vi "sv_Get Continuous Swept Sine Settings (1 Ch).vi"(8 "error in (no error)":errorcluster, 10 "chirp settings in":T1 {"frequency slope" format="%.2f"; "prefix len [samples]"."fractional" format="%.2p"; "initial states"."elapsed time [s]" format="%.2f"; "initial states"."phase [rad]" format="%.2f"; "initial states"."frequency [Hz]" format="%.2f"; "sampling info"."chirp duration [s]" format="%.2f"; "sampling info"."Fs" format="%.2p"; "frequency range"."stop (Hz)" format="%.2f"; "frequency range"."start (Hz)" format="%.2f"; "amplitude" format="%.2f"}, 11 "waveform":waveform(dbl)) -> (0 "error out":errorcluster, 2 "chirp settings out":T1 {"frequency slope" format="%.2f"; "prefix len [samples]"."fractional" format="%.2p"; "initial states"."elapsed time [s]" format="%.2f"; "initial states"."phase [rad]" format="%.2f"; "initial states"."frequency [Hz]" format="%.2f"; "sampling info"."chirp duration [s]" format="%.2f"; "sampling info"."Fs" format="%.2p"; "frequency range"."stop (Hz)" format="%.2f"; "frequency range"."start (Hz)" format="%.2f"; "amplitude" format="%.2f"}, 3 "same waveform":waveform(dbl))   [LabVIEW 2017]
uses:
  <vilib>/addons/_NISVFA/_Generation/subVIs/sv_Chirp Settings.ctl
  <vilib>/addons/_NISVFA/_Generation/SoundVib_Generation.lvlib
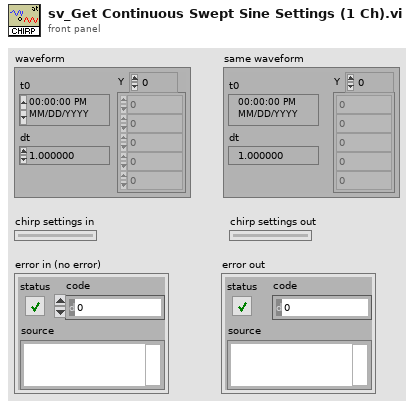
[diagram p1: front panel]
types:
  T1 = typedef "SoundVib_Generation.lvlib/sv_Chirp Settings.ctl" = cluster{"amplitude":dbl, "frequency range":cluster{"start (Hz)":dbl, "stop (Hz)":dbl, "frequency spacing":enum16{"Linear", "Logarithmic"}}, "sampling info":cluster{"Fs":dbl, "chirp duration [s]":dbl}, "initial states":cluster{"frequency [Hz]":dbl, "phase [rad]":dbl, "elapsed time [s]":dbl}, "frequency slope":dbl, "maximum harmonic":i32, "prefix len [samples]":cluster{"integer":u32, "fractional":dbl}}
  T2 = enum16{"ChirpAmplitude", "ChirpStartFrequency", "ChirpStopFrequency", "ChirpFrequencySpacing", "ChirpSamplingRate", "ChirpDuration", "ChirpCurrentFrequency", "ChirpCurrentPhase", "ChirpCurrentTime", "ChirpSlope", "ChirpMaxHarmonic", "ChirpPrefixInteger", "ChirpPrefixFractional"}
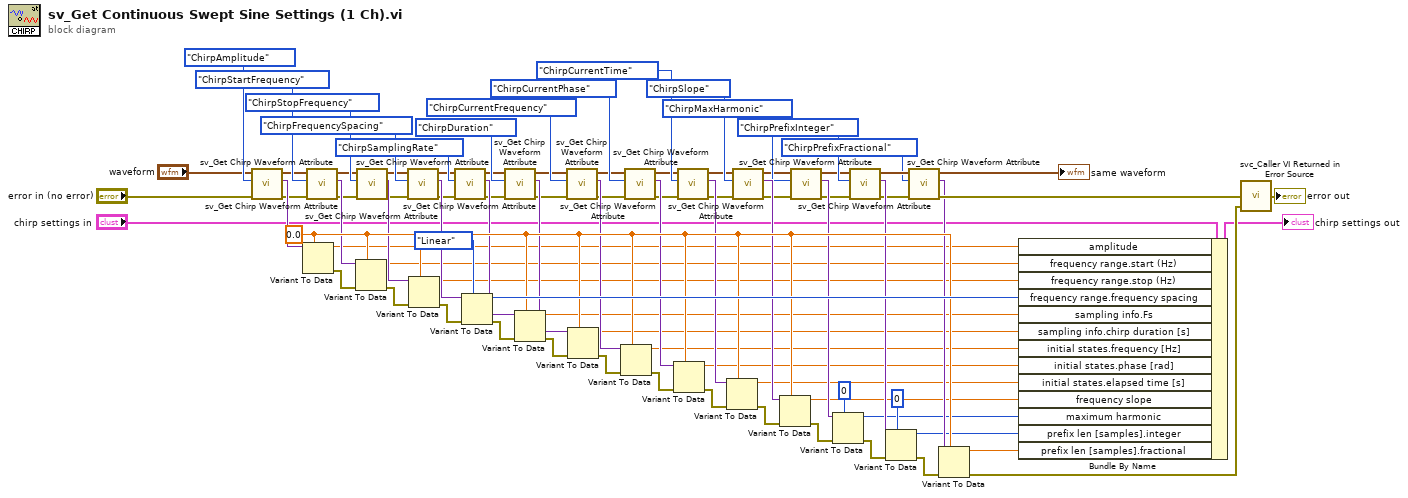
[diagram p0: block diagram]
diagram:
  w68 = 0.0 ("amplitude")
  n1 = call <vilib>:"sv_Get Chirp Waveform Attribute.vi"("error in (no error)"="error in (no error)", "chirp attributes"=T2."ChirpAmplitude", "chirp signal"="waveform") -> ("error out"=w6:errorcluster, "attribute value"=w41:variant, "chirp signal out"=w5:waveform(dbl))  [unwired: 6 in]
  n2 = Variant To Data(type=w68, Variant=w41) -> (data=w42:dbl, error out=w73:errorcluster)  [unwired: 1 in]
  n3 = call <vilib>:"sv_Get Chirp Waveform Attribute.vi"("error in (no error)"=w6, "chirp attributes"=T2."ChirpStartFrequency", "chirp signal"=w5) -> ("error out"=w8:errorcluster, "attribute value"=w43:variant, "chirp signal out"=w9:waveform(dbl))  [unwired: 6 in]
  n4 = Variant To Data(error in=w73, type=w68, Variant=w43) -> (data=w44:dbl, error out=w71:errorcluster)
  n5 = call <vilib>:"sv_Get Chirp Waveform Attribute.vi"("error in (no error)"=w8, "chirp attributes"=T2."ChirpStopFrequency", "chirp signal"=w9) -> ("error out"=w12:errorcluster, "attribute value"=w45:variant, "chirp signal out"=w11:waveform(dbl))  [unwired: 6 in]
  n6 = call <vilib>:"sv_Get Chirp Waveform Attribute.vi"("error in (no error)"=w12, "chirp attributes"=T2."ChirpFrequencySpacing", "chirp signal"=w11) -> ("error out"=w15:errorcluster, "attribute value"=w47:variant, "chirp signal out"=w14:waveform(dbl))  [unwired: 6 in]
  n7 = Variant To Data(error in=w71, type=w68, Variant=w45) -> (data=w46:dbl, error out=w72:errorcluster)
  n8 = call <vilib>:"sv_Get Chirp Waveform Attribute.vi"("error in (no error)"=w15, "chirp attributes"=T2."ChirpSamplingRate", "chirp signal"=w14) -> ("error out"=w17:errorcluster, "attribute value"=w48:variant, "chirp signal out"=w18:waveform(dbl))  [unwired: 6 in]
  n9 = Variant To Data(error in=w72, type=enum16{"Linear", "Logarithmic"}."Linear" ("frequency range.frequency spacing"), Variant=w47) -> (data=w87:enum16{"Linear", "Logarithmic"}, error out=w74:errorcluster)
  n10 = call <vilib>:"sv_Get Chirp Waveform Attribute.vi"("error in (no error)"=w17, "chirp attributes"=T2."ChirpDuration", "chirp signal"=w18) -> ("error out"=w20:errorcluster, "attribute value"=w50:variant, "chirp signal out"=w21:waveform(dbl))  [unwired: 6 in]
  n11 = Variant To Data(error in=w74, type=w68, Variant=w48) -> (data=w49:dbl, error out=w75:errorcluster)
  n12 = call <vilib>:"sv_Get Chirp Waveform Attribute.vi"("error in (no error)"=w20, "chirp attributes"=T2."ChirpCurrentFrequency", "chirp signal"=w21) -> ("error out"=w24:errorcluster, "attribute value"=w52:variant, "chirp signal out"=w23:waveform(dbl))  [unwired: 6 in]
  n13 = Variant To Data(error in=w75, type=w68, Variant=w50) -> (data=w51:dbl, error out=w76:errorcluster)
  n14 = Variant To Data(error in=w76, type=w68, Variant=w52) -> (data=w53:dbl, error out=w77:errorcluster)
  n15 = call <vilib>:"sv_Get Chirp Waveform Attribute.vi"("error in (no error)"=w24, "chirp attributes"=T2."ChirpCurrentPhase", "chirp signal"=w23) -> ("error out"=w26:errorcluster, "attribute value"=w54:variant, "chirp signal out"=w27:waveform(dbl))  [unwired: 6 in]
  n16 = Variant To Data(error in=w77, type=w68, Variant=w54) -> (data=w55:dbl, error out=w78:errorcluster)
  n17 = call <vilib>:"sv_Get Chirp Waveform Attribute.vi"("error in (no error)"=w26, "chirp attributes"=T2."ChirpCurrentTime", "chirp signal"=w27) -> ("error out"=w29:errorcluster, "attribute value"=w56:variant, "chirp signal out"=w30:waveform(dbl))  [unwired: 6 in]
  n18 = Variant To Data(error in=w78, type=w68, Variant=w56) -> (data=w57:dbl, error out=w79:errorcluster)
  n19 = call <vilib>:"sv_Get Chirp Waveform Attribute.vi"("error in (no error)"=w29, "chirp attributes"=T2."ChirpSlope", "chirp signal"=w30) -> ("error out"=w33:errorcluster, "attribute value"=w58:variant, "chirp signal out"=w32:waveform(dbl))  [unwired: 6 in]
  n20 = Variant To Data(error in=w79, type=w68, Variant=w58) -> (data=w59:dbl, error out=w80:errorcluster)
  n21 = call <vilib>:"sv_Get Chirp Waveform Attribute.vi"("error in (no error)"=w33, "chirp attributes"=T2."ChirpMaxHarmonic", "chirp signal"=w32) -> ("error out"=w36:errorcluster, "attribute value"=w60:variant, "chirp signal out"=w35:waveform(dbl))  [unwired: 6 in]
  n22 = Variant To Data(error in=w80, type=0 ("maximum harmonic"), Variant=w60) -> (data=w62:i32, error out=w81:errorcluster)
  n23 = call <vilib>:"sv_Get Chirp Waveform Attribute.vi"("error in (no error)"=w36, "chirp attributes"=T2."ChirpPrefixInteger", "chirp signal"=w35) -> ("error out"=w40:errorcluster, "attribute value"=w63:variant, "chirp signal out"=w39:waveform(dbl))  [unwired: 6 in]
  n24 = Variant To Data(error in=w81, type=u32 0 ("prefix len [samples].integer"), Variant=w63) -> (data=w65:u32, error out=w82:errorcluster)
  n25 = call <vilib>:"sv_Get Chirp Waveform Attribute.vi"("error in (no error)"=w40, "chirp attributes"=T2."ChirpPrefixFractional", "chirp signal"=w39) -> ("error out"=w84:errorcluster, "attribute value"=w67:variant, "chirp signal out"=→"same waveform":waveform(dbl))  [unwired: 6 in]
  n26 = Variant To Data(error in=w82, type=w68, Variant=w67) -> (data=w66:dbl, error out=w83:errorcluster)
  n27 = Bundle By Name(cluster="chirp settings in", "amplitude"=w42, "frequency range.start (Hz)"=w44, "frequency range.stop (Hz)"=w46, "frequency range.frequency spacing"=w87, "sampling info.Fs"=w49, "sampling info.chirp duration [s]"=w51, "initial states.frequency [Hz]"=w53, "initial states.phase [rad]"=w55, "initial states.elapsed time [s]"=w57, "frequency slope"=w59, "maximum harmonic"=w62, "prefix len [samples].integer"=w65, "prefix len [samples].fractional"=w66) -> (→"chirp settings out":T1)
  n28 = call <vilib>:"svc_Caller VI Returned in Error Source.vi"("warning input to caller"=w83, "error in (no error)"=w84) -> ("error out"=→"error out":errorcluster)  [unwired: 3 in]
